vi "M prepare for Solar.vi"(11 "EV3 in":T1) -> (3 "EV3 out":T1)   [LabVIEW 2016]
uses:
  <vilib>/NXT/Subs/LVHSConnector.ctl
  <vilib>/NXT/LegoClasses/BrickReference/BrickReference.lvclass
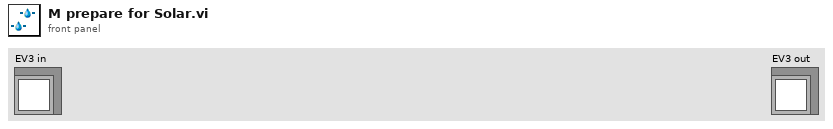
[diagram p1: front panel]
types:
  T1 = typedef "LVHSConnector.ctl" = refnum<class "BrickReference.lvclass">
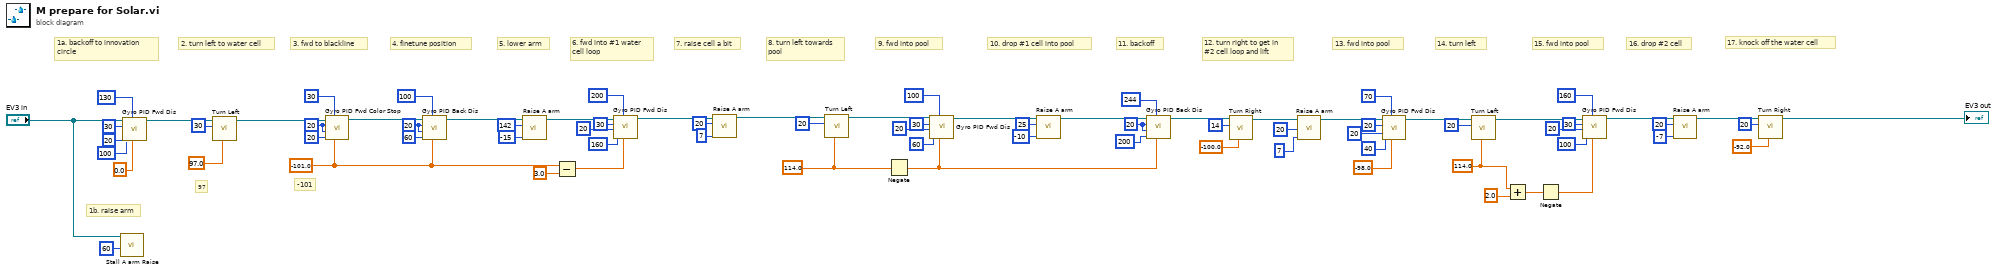
[diagram p0: block diagram]
diagram:
  w7 = sgl 114.0 ("Turning angle")
  w32 = sgl 114.0 ("Turning angle")
  w41 = 20 ("Max. speed")
  w60 = 20 ("Max. speed")
  w38 = sgl -101.0 ("Target angle")
  w64 = 20 ("Max. speed")
  # "17. knock off the water cell"
  # "97"
  # "-101"
  # "16. drop #2 cell"
  # "15. fwd into pool"
  # "14. turn left"
  # "13. fwd into pool"
  # "12. turn right to get in\n#2 cell loop and lift"
  # "8. turn left towards\npool"
  # "11. backoff"
  # "9. fwd into pool"
  # "6. fwd into #1 water\ncell loop"
  # "4. finetune position"
  # "3. fwd to blackline"
  # "1b. raise arm"
  # "10. drop #1 cell into pool"
  # "7. raise cell a bit"
  # "5. lower arm"
  # "2. turn left to water cell"
  # "1a. backoff to innovation\ncircle"
  n1 = call "Stall A arm Raise.vi"("Power"=i8 60, "NXT/EV3"="EV3 in") -> ()  [unwired: 9 in, 1 out]
  n2 = call "Gyro PID Fwd Dis.vi"("Target angle"=sgl 0.0, "Threshold to stop"=130, "Threshold to slow"=100, "Min. speed"=20, "Max. speed"=30, "EV3 in"="EV3 in") -> ("EV3 out"=w73:T1)  [unwired: 5 in]
  n3 = call "Turn Left.vi"("Turning angle"=sgl 97.0, "Motor B (right)"=i8 30, "EV3 in"=w73) -> ("EV3 out"=w66:T1)  [unwired: 8 in]
  n4 = call "Gyro PID Fwd Color Stop.vi"("Target angle"=w38, "Threshold to Color"=30, "Threshold to slow"=20, "Min. speed"=w64, "Max. speed"=w64, "EV3 in"=w66) -> ("EV3 out"=w62:T1)  [unwired: 5 in]
  n5 = call "Gyro PID Back Dis.vi"("Target angle"=w38, "Threshold to stop"=100, "Threshold to slow"=60, "Min. speed"=w60, "Max. speed"=w60, "EV3 in"=w62) -> ("EV3 out"=w58:T1)  [unwired: 5 in]
  n6 = call "Raise A arm.vi"("Power"=i8 -15, "Rotation"=142, "EV3 in"=w58) -> ("EV3 out"=w57:T1)  [unwired: 8 in]
  n7 = Subtract(x=w38, y=sgl 3.0) -> (x-y=w37:sgl)
  n8 = call "Gyro PID Fwd Dis.vi"("Target angle"=w37, "Threshold to stop"=200, "Threshold to slow"=160, "Min. speed"=20, "Max. speed"=30, "EV3 in"=w57) -> ("EV3 out"=w52:T1)  [unwired: 5 in]
  n9 = call "Raise A arm.vi"("Power"=i8 7, "Rotation"=20, "EV3 in"=w52) -> ("EV3 out"=w35:T1)  [unwired: 8 in]
  n10 = call "Turn Left.vi"("Turning angle"=w32, "Motor B (right)"=i8 20, "EV3 in"=w35) -> ("EV3 out"=w34:T1)  [unwired: 8 in]
  n11 = Negate(x=w32) -> (-x=w31:sgl)
  n12 = call "Gyro PID Fwd Dis.vi"("Target angle"=w31, "Threshold to stop"=100, "Threshold to slow"=60, "Min. speed"=20, "Max. speed"=30, "EV3 in"=w34) -> ("EV3 out"=w44:T1)  [unwired: 5 in]
  n13 = call "Raise A arm.vi"("Power"=i8 -10, "Rotation"=25, "EV3 in"=w44) -> ("EV3 out"=w39:T1)  [unwired: 8 in]
  n14 = call "Gyro PID Back Dis.vi"("Target angle"=w31, "Threshold to stop"=244, "Threshold to slow"=200, "Min. speed"=w41, "Max. speed"=w41, "EV3 in"=w39) -> ("EV3 out"=w20:T1)  [unwired: 5 in]
  n15 = call "Turn Right.vi"("Turning angle"=sgl -100.0, "Motor B (right)"=i8 14, "EV3 in"=w20) -> ("EV3 out"=w18:T1)  [unwired: 8 in]
  n16 = call "Raise A arm.vi"("Power"=i8 7, "Rotation"=20, "EV3 in"=w18) -> ("EV3 out"=w14:T1)  [unwired: 8 in]
  n17 = call "Gyro PID Fwd Dis.vi"("Target angle"=sgl -98.0, "Threshold to stop"=70, "Threshold to slow"=40, "Min. speed"=20, "Max. speed"=20, "EV3 in"=w14) -> ("EV3 out"=w13:T1)  [unwired: 5 in]
  n18 = call "Turn Left.vi"("Turning angle"=w7, "Motor B (right)"=i8 20, "EV3 in"=w13) -> ("EV3 out"=w8:T1)  [unwired: 8 in]
  n19 = Add(x=w7, y=sgl 2.0) -> (x+y=w6:sgl)
  n20 = Negate(x=w6) -> (-x=w5:sgl)
  n21 = call "Gyro PID Fwd Dis.vi"("Target angle"=w5, "Threshold to stop"=160, "Threshold to slow"=100, "Min. speed"=20, "Max. speed"=30, "EV3 in"=w8) -> ("EV3 out"=w4:T1)  [unwired: 5 in]
  n22 = call "Raise A arm.vi"("Power"=i8 -7, "Rotation"=20, "EV3 in"=w4) -> ("EV3 out"=w23:T1)  [unwired: 8 in]
  n23 = call "Turn Right.vi"("Turning angle"=sgl -92.0, "Motor B (right)"=i8 20, "EV3 in"=w23) -> ("EV3 out"=→"EV3 out":T1)  [unwired: 8 in]
